vi "Resume Process.vi"(8 "error in (no error)":errorcluster, 11 "Process Model in":refnum<class "Process Model.lvclass">) -> (0 "error out":errorcluster, 3 "Process Model out":refnum<class "Process Model.lvclass">)   [LabVIEW 2019, in "Process Model.lvclass"]
uses:
  <vilib>/gpm_packages/@cs/Car-wash/Source/Process Model/Process Model.lvclass
  C:/Program Files/National Instruments/LabVIEW 2019/vi.lib/ActorFramework/Actor/Actor.lvclass
  <vilib>/ActorFramework/Message Enqueuer/Message Enqueuer.lvclass
  <vilib>/gpm_packages/@cs/Car-wash/Source/Process Model/Process Model.lvclass/Process Model.ctl
  <vilib>/ActorFramework/Message Enqueuer/Message Enqueuer.lvclass/Message Enqueuer.ctl
  <vilib>/ActorFramework/Actor/Actor.lvclass/Actor.ctl
  <vilib>/ActorFramework/Message Enqueuer/Enqueue.vi
  <vilib>/ActorFramework/Message Enqueuer/Init from Existing Queue.vi
  <vilib>/gpm_packages/@cs/Car-wash/Source/iProcess Step Model/iProcess Step Model Messages/Resume Msg/Resume Msg.lvclass
  C:/Program Files/National Instruments/LabVIEW 2019/vi.lib/ActorFramework/Message/Message.lvclass
  <vilib>/gpm_packages/@cs/Car-wash/Source/iProcess Model/iProcess Model Messages/Execute Process Msg/Execute Process Step Msg.lvclass
  <vilib>/ActorFramework/Message Priority Queue/Priority Enqueue.vi
  <vilib>/ActorFramework/Actor/Actor.lvclass
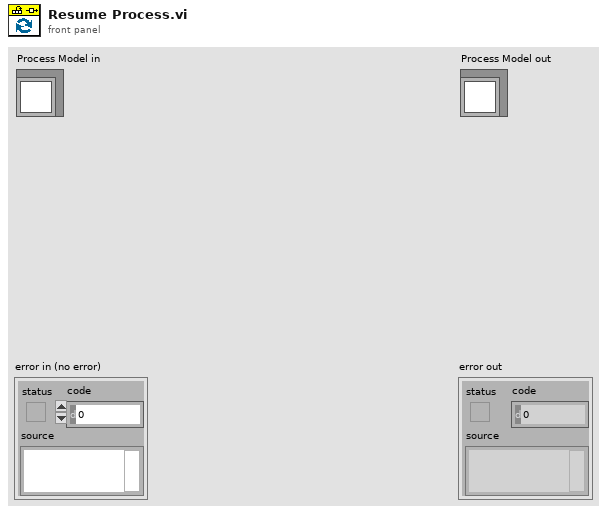
[diagram p1: front panel]
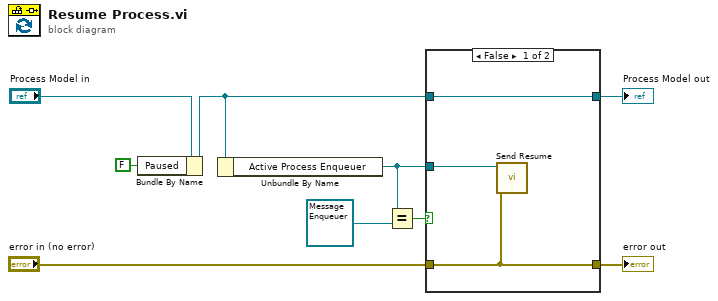
[diagram p0: block diagram]
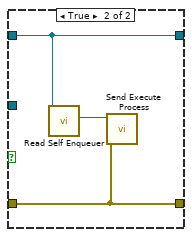
[diagram p2: hidden frame]
diagram:
  n1 = Bundle By Name(cluster="Process Model in", "Paused"=FALSE) -> (w4:refnum<class "Process Model.lvclass">)
  n2 = Unbundle By Name(w4) -> ("Active Process Enqueuer"=w7:refnum<class "Message Enqueuer.lvclass">)
  n3 = Equal?(x=w7, y=refnum<class "Message Enqueuer.lvclass"> refnum) -> (x = y?=w5:bool)
  n4 = case shown="False" w5 {
    tunnel: w7 -> [w12 _]
    tunnel: [w11 w14] -> w3
    tunnel: w4 -> [w11 w14]
    tunnel: [w10 w13] -> w1
    tunnel: "error in (no error)" -> [w10 w13]
    frame False {
      n5 = call <vilib>:"Send Resume.vi"("error in (no error)"=w10, "Message Enqueuer"=w12) -> ()  [unwired: 8 in, 2 out]
    }
    frame True {
      n6 = call <vilib>:"Read Self Enqueuer.vi"("Actor"=w14) -> ("Self Enqueuer"=w15:refnum<class "Message Enqueuer.lvclass">)  [unwired: 10 in]
      n7 = call <vilib>:"Send Execute Process.vi"("error in (no error)"=w13, "Message Enqueuer"=w15) -> ()  [unwired: 8 in, 2 out]
    }
  }
  "error out" <- w1
  "Process Model out" <- w3
